vi "Example Cluster Bundler and Class.vi"() -> ()   [LabVIEW 2018]
uses:
  Example Translator Vis/Example Vector of Floats.ctl
panel:
  out "Cluster":cluster{sgl, sgl, sgl}
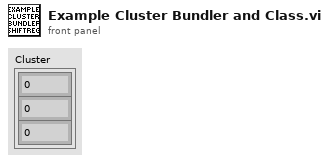
[diagram p1: front panel]
types:
  T1 = typedef "Example Vector of Floats.ctl" = cluster{sgl, sgl, sgl}
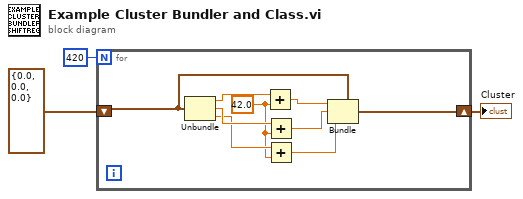
[diagram p0: block diagram]
diagram:
  n1 = for {
    N: 420 -> [_]
    shift-right: [w4] -> w2
    shift-left: T1 {0.0, 0.0, 0.0} -> [w12]
    w8 = sgl 42.0 ("y")
    n2 = Unbundle(w12) -> (w11:sgl, w10:sgl, w9:sgl)
    n3 = Add(x=w11, y=w8) -> (x+y=w7:sgl)
    n4 = Add(x=w10, y=w8) -> (x+y=w6:sgl)
    n5 = Add(x=w9, y=w8) -> (x+y=w5:sgl)
    n6 = Bundle(cluster=w12, w7, w6, w5) -> (w4:T1)
  }
  "Cluster" <- w2
